vi "Array-Parse From String.vi"(7 "String":string, 11 "error in (no error)":errorcluster) -> (8 "Array":dbl[](array[numeric]), 15 "error out":errorcluster)   [LabVIEW 2020]
uses:
  <vilib>/regexp/Match Regular Expression.xnode
  <vilib>/gmath/NI_Gmath.lvlib
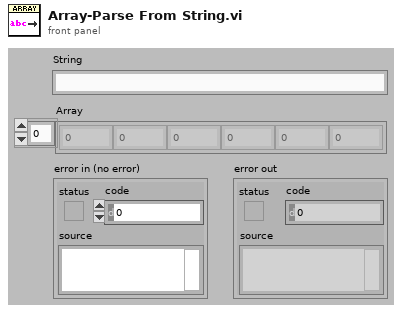
[diagram p1: front panel]
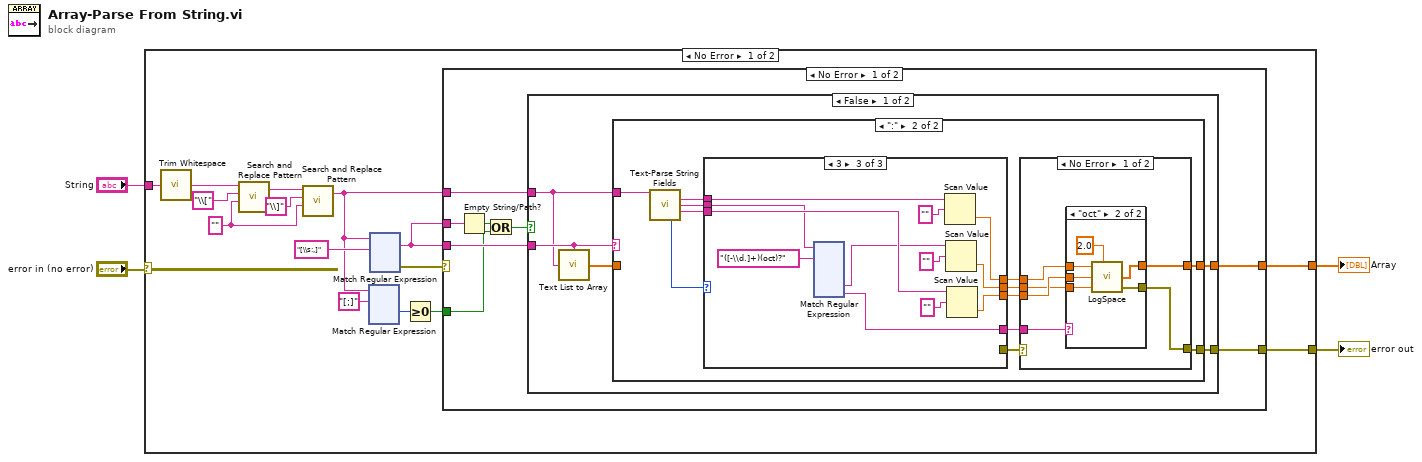
[diagram p0: block diagram]
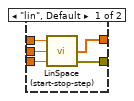
[diagram p3: hidden frame]
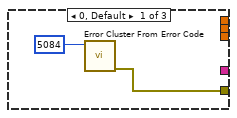
[diagram p5: hidden frame]
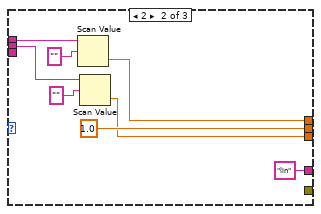
[diagram p6: hidden frame]
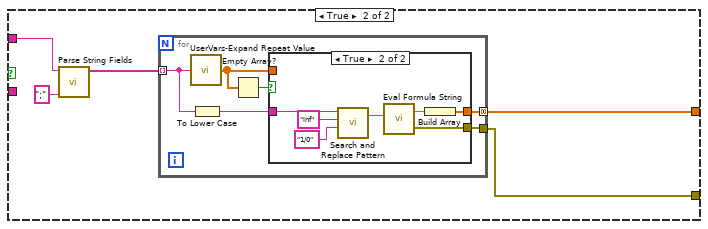
[diagram p7: hidden frame]
diagram:
  n1 = case shown="No Error" "error in (no error)" {
    selector: "error in (no error)" -> [_ w445]
    tunnel: [w15 w445] -> w3
    tunnel: "String" -> [w6 _]
    tunnel: [w16 _] -> w1
    frame No Error {
      w12 = "" ("replace string (\"\")")
      n2 = call <vilib>:"Trim Whitespace.vi"("string"=w6) -> ("trimmed string"=w5:string)  [unwired: 1 in]
      n3 = call <vilib>:"Search and Replace Pattern.vi"("string"=w5, "regular expression (\"\")"="\\[" ("regular expression (\"\")"), "replace string (\"\")"=w12) -> ("result string"=w11:string)  [unwired: 2 in, 1 out]
      n4 = call <vilib>:"Search and Replace Pattern.vi"("string"=w11, "regular expression (\"\")"="\\]" ("regular expression (\"\")"), "replace string (\"\")"=w12) -> ("result string"=w10:string)  [unwired: 2 in, 1 out]
      n5 = xnode "Match Regular Expression"("input string"=w10, "regular expression"="[;]") -> ("offset past match"=w8:i32)  [unwired: 4 in, 4 out]
      n6 = xnode "Match Regular Expression"("input string"=w10, "regular expression"="[\\s:,]") -> ("whole match"=w17:string, "error out"=w18:errorcluster)  [unwired: 4 in, 3 out]
      n7 = Greater Or Equal To 0?(x=w8) -> (x >= 0?=w7:bool)
      n8 = case shown="No Error" w18 {
        selector: w18 -> [_ w333]
        tunnel: w17 -> [w138 _]
        tunnel: w17 -> [w136 _]
        tunnel: w10 -> [w135 _]
        tunnel: [w134 _] -> w16
        tunnel: [w133 w333] -> w15
        tunnel: w7 -> [w131 _]
        frame No Error {
          n9 = Empty String/Path?(string/path=w138) -> (empty?=w137:bool)
          n10 = Or(x=w137, y=w131) -> (x .or. y?=w132:bool)
          n11 = case shown="False" w132 {
            tunnel: w136 -> [w142 _]
            tunnel: w135 -> [w139 w317]
            tunnel: [w141 w315] -> w134
            tunnel: [w140 w318] -> w133
            frame False {
              n12 = call "Text List to Array.vi"("delimiter (;)"=w142, "text list"=w139) -> ("array"=w143:dbl[])  [unwired: 2 in]
              n13 = case shown="\":\"" w142 {
                tunnel: w143 -> [w144 _]
                tunnel: [w144 w153] -> w141
                tunnel: [_ w152] -> w140
                tunnel: w139 -> [_ w150]
                frame "False", Default {
                }
                frame ":" {
                  n14 = call "Text-Parse String Fields.vi"("String"=w150) -> ("element"=w148:string, "element 2"=w147:string, "element 3"=w146:string, "Number of fields"=w149:u32)  [unwired: 9 in, 2 out]
                  n15 = case shown="3" w149 {
                    tunnel: [_ w178 w192] -> w156
                    tunnel: [_ w179 w190] -> w155
                    tunnel: [_ 1.0 w186] -> w154
                    tunnel: [w176 _ _] -> w151
                    tunnel: w148 -> [_ w182 w193]
                    tunnel: w147 -> [_ w180 w188]
                    tunnel: w146 -> [_ _ w191]
                    tunnel: [_ "lin" ("submatch 2") w185] -> w145
                    frame 0, Default {
                      n16 = call <vilib>:"Error Cluster From Error Code.vi"("error code (0)"=5084) -> ("error out"=w176:errorcluster)  [unwired: 8 in]
                    }
                    frame 2 {
                      n17 = Scan Value(string=w182, format string="") -> (value=w178:dbl)  [unwired: 1 in, 1 out]
                      n18 = Scan Value(string=w180, format string="") -> (value=w179:dbl)  [unwired: 1 in, 1 out]
                    }
                    frame 3 {
                      n19 = xnode "Match Regular Expression"("input string"=w188, "regular expression"="([-\\d.]+)(oct)?") -> ("submatch 1"=w187:string, "submatch 2"=w185:string)  [unwired: 4 in, 5 out]
                      n20 = Scan Value(string=w193, format string="") -> (value=w192:dbl)  [unwired: 1 in, 1 out]
                      n21 = Scan Value(string=w187, format string="") -> (value=w186:dbl)  [unwired: 1 in, 1 out]
                      n22 = Scan Value(string=w191, format string="") -> (value=w190:dbl)  [unwired: 1 in, 1 out]
                    }
                  }
                  n23 = case shown="No Error" w151 {
                    selector: w151 -> [_ w174]
                    tunnel: w156 -> [w162 _]
                    tunnel: w155 -> [w161 _]
                    tunnel: w154 -> [w160 _]
                    tunnel: [w159 _] -> w153
                    tunnel: [w158 w174] -> w152
                    tunnel: w145 -> [w157 _]
                    frame No Error {
                      n24 = case shown="\"oct\"" w157 {
                        tunnel: w162 -> [w167 w173]
                        tunnel: w161 -> [w166 w172]
                        tunnel: w160 -> [w165 w171]
                        tunnel: [w164 w170] -> w159
                        tunnel: [w163 w168] -> w158
                        frame "lin", Default {
                          n25 = call "LinSpace (start-stop-step).vi"("Step"=w165, "Stop"=w166, "Start"=w167) -> ("error out"=w163:errorcluster, "Array"=w164:dbl[])  [unwired: 1 in]
                        }
                        frame "oct" {
                          n26 = call "LogSpace.vi"("Start"=w173, "Base"=2.0, "Stop"=w172, "Step"=w171) -> ("Array"=w170:dbl[], "error out"=w168:errorcluster)  [unwired: 2 in]
                        }
                      }
                    }
                    frame Error {
                    }
                  }
                }
              }
            }
            frame True {
              n27 = call "Parse String Fields.vi"("Separator"=";", "String"=w317) -> ("Fields"=w314:string[])  [unwired: 8 in, 1 out]
              n28 = for {
                tunnel: [w324] -> w315 mode=concatenating
                tunnel: [w323] -> w318
                tunnel: w314 -> [w320] mode=indexing
                n29 = call "UserVars-Expand Repeat Value.vi"("Expression"=w320) -> ("repeated values"=w322:dbl[])  [unwired: 14 in]
                n30 = To Lower Case(string=w320) -> (all lower case string=w319:string)
                n31 = Empty Array?(array=w322) -> (empty?=w321:bool)
                n32 = case shown="True" w321 {
                  tunnel: [w325 w330] -> w324
                  tunnel: [_ w331] -> w323
                  tunnel: w322 -> [w325 _]
                  tunnel: w319 -> [_ w329]
                  frame False {
                  }
                  frame True {
                    n33 = call <vilib>:"Search and Replace Pattern.vi"("string"=w329, "regular expression (\"\")"="inf" ("regular expression (\"\")"), "replace string (\"\")"="1/0" ("replace string (\"\")")) -> ("result string"=w328:string)  [unwired: 2 in, 1 out]
                    n34 = call <vilib>:"Eval Formula String.vi"("formula"=w328) -> ("error out"=w331:errorcluster, "y value"=w332:dbl)  [unwired: 1 in]
                    n35 = Build Array(w332) -> (w330:dbl[])
                  }
                }
              }
            }
          }
        }
        frame Error {
        }
      }
    }
    frame Error {
    }
  }
  "error out" <- w3
  "Array" <- w1
